vi "Graphics-Draw Bracket (Picture).vi"(0 "picture in":picture, 7 "rect":T1, 11 "point left":bool, 12 "color(black)":u32(colorbox)=16711680, 13 "pen":T2) -> (4 "picture out":picture)   [LabVIEW 2020]
uses:
  <vilib>/Utility/miscctls.llb/LVRectTypeDef.ctl
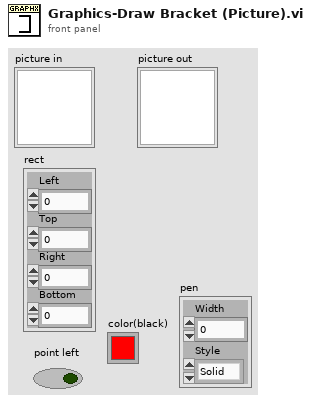
[diagram p1: front panel]
types:
  T1 = typedef "LVRectTypeDef.ctl" = cluster{"Left":i16, "Top":i16, "Right":i16, "Bottom":i16}
  T2 = cluster{"Width":u16, "Style":enum32{"Solid", "Dash", "Dot", "DashDot", "DashDotDot"}}
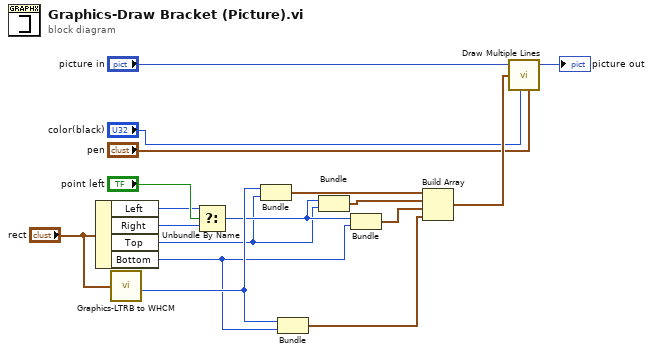
[diagram p0: block diagram]
diagram:
  n1 = Unbundle By Name("rect") -> ("Left"=w13:i16, "Right"=w14:i16, "Top"=w9:i16, "Bottom"=w11:i16)
  n2 = call "Graphics-LTRB to WHCM.vi"("LTRB"="rect") -> ("Center"=w12:i16)  [unwired: 4 in, 3 out]
  n3 = Select(t=w13, s="point left", f=w14) -> (s? t:f=w10:i16)
  n4 = Bundle("Center"=w12, "Top"=w9) -> (w8:cluster{"Center":i16, "Top":i16})  [unwired: 1 in]
  n5 = Bundle("Center"=w12, "Bottom"=w11) -> (w5:cluster{"Center":i16, "Bottom":i16})  [unwired: 1 in]
  n6 = Bundle("Right"=w10, "Top"=w9) -> (w7:cluster{"Right":i16, "Top":i16})  [unwired: 1 in]
  n7 = Bundle("Right"=w10, "Bottom"=w11) -> (w6:cluster{"Right":i16, "Bottom":i16})  [unwired: 1 in]
  n8 = Build Array(w8, w7, w6, w5) -> (w4:cluster{"Center":i16, "Bottom":i16}[])
  n9 = call <vilib>:"Draw Multiple Lines.vi"("picture"="picture in", "line endpoints"=w4, "color(black)"="color(black)", "pen"="pen") -> ("new picture"=→"picture out":picture)  [unwired: 5 in]
